vi "Message for Default Reset Import.vi"(9 "New Value (Default)":string[](array[string]), 10 "Old Value":string[](array[string]), 11 "Key":string[](array[string])) -> ()   [LabVIEW 2020, in "ConditionalDeactivation.lvlib"]
uses:
  ConditionalDeactivation.lvlib
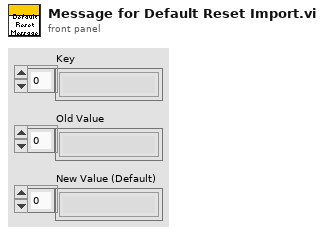
[diagram p1: front panel]
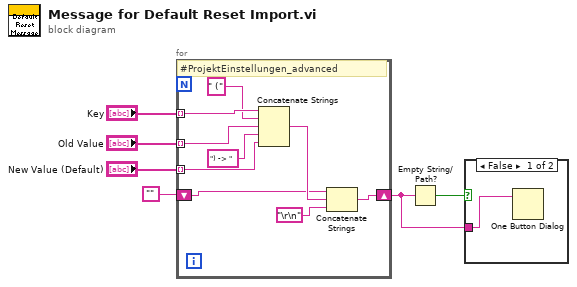
[diagram p0: block diagram]
diagram:
  n1 = for {
    tunnel: "Key" -> [w15] mode=indexing
    tunnel: "New Value (Default)" -> [w11] mode=indexing
    tunnel: "Old Value" -> [w13] mode=indexing
    shift-right: [w9] -> w1
    shift-left: "" -> [w8]
    # "#ProjektEinstellungen_advanced"
    n2 = Concatenate Strings(w15, " (" ("String"), w13, ") -> " ("String"), w11) -> (w10:string)
    n3 = Concatenate Strings(w8, w10, "\r\n") -> (w9:string)
  }
  n4 = Empty String/Path?(string/path=w1) -> (empty?=w3:bool)
  n5 = case shown="False" w3 {
    tunnel: w1 -> [w16 _]
    frame False {
      n6 = One Button Dialog(message=w16) -> ()  [unwired: 1 in, 1 out]
    }
    frame True {
    }
  }
